vi "Configure Calib Factor (IO).vi"(0 "VISA resource name":refnum<visa-resource-name>, 5 "Channel (0001)":string="0001", 7 "Correct Factor (ON)":bool=TRUE, 9 "Calibration Correction":T1(array[cluster]) {"Sensor Correction Factor" min=-999999 max=999999 step=1; "Instrument Correction Factor" min=-999999 max=999999 step=1; "Uncorrected Value" min=-999999 max=999999 step=1}, 11 "error in (no error)":errorcluster) -> (4 "VISA resource name out":refnum<visa-resource-name>, 6 "Channel":string, 15 "error out":errorcluster)   [LabVIEW 2020, in "Yokogawa GX Series.lvlib"]
doc: "Sets the calibration correction(Correction Factor) for AI channels.\n\nCommand: SCalibIO"
uses:
  <instrlib>/Yokogawa GX Series/Yokogawa GX Series.lvlib
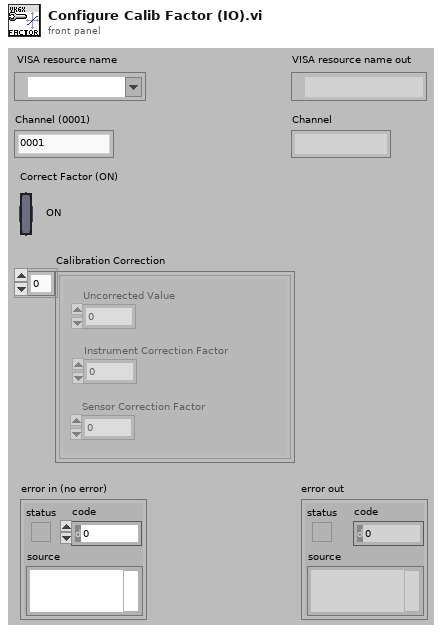
[diagram p1: front panel]
types:
  T1 = cluster{"Uncorrected Value":i32, "Instrument Correction Factor":i32, "Sensor Correction Factor":i32}[]
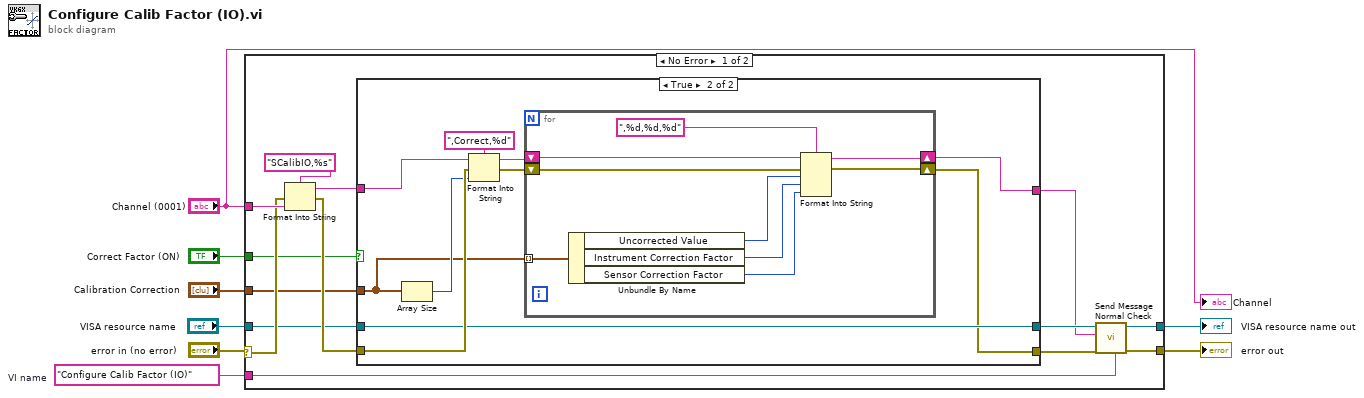
[diagram p0: block diagram]
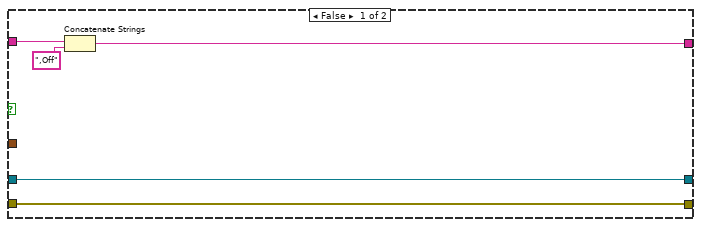
[diagram p2: hidden frame]
diagram:
  w8 = "Configure Calib Factor (IO)"  # VI name
  n1 = case shown="No Error" "error in (no error)" {
    selector: "error in (no error)" -> [w15 w47]
    tunnel: w8 -> [w22 _]
    tunnel: [w21 w48] -> w7
    tunnel: [w20 w47] -> w6
    tunnel: "VISA resource name" -> [w14 w48]
    tunnel: "Channel (0001)" -> [w16 _]
    tunnel: "Correct Factor (ON)" -> [w11 _]
    tunnel: "Calibration Correction" -> [w10 _]
    frame No Error {
      n2 = Format Into String(format string="SCalibIO,%s", error in=w15, w16) -> (resulting string=w18:string, error out=w17:errorcluster)  [unwired: 1 in]
      n3 = case shown="True" w11 {
        tunnel: w18 -> [w27 w29]
        tunnel: [w25 w33] -> w9
        tunnel: w17 -> [w23 w36]
        tunnel: w14 -> [w24 w32]
        tunnel: [w24 w32] -> w13
        tunnel: [w23 w31] -> w12
        tunnel: w10 -> [_ w28]
        frame False {
          n4 = Concatenate Strings(w27, ",Off") -> (w25:string)
        }
        frame True {
          n5 = Array Size(array=w28) -> (size(s)=w30:i32)
          n6 = Format Into String(format string=",Correct,%d", initial string=w29, error in=w36, w30) -> (resulting string=w35:string, error out=w34:errorcluster)
          n7 = for {
            shift-right: [w43] -> w33
            shift-left: w35 -> [w46]
            shift-right: [w44] -> w31
            shift-left: w34 -> [w45]
            tunnel: w28 -> [w40] mode=indexing
            n8 = Unbundle By Name(w40) -> ("Uncorrected Value"=w41:i32, "Instrument Correction Factor"=w39:i32, "Sensor Correction Factor"=w38:i32)
            n9 = Format Into String(format string=",%d,%d,%d", initial string=w46, error in=w45, w41, w39, w38) -> (resulting string=w43:string, error out=w44:errorcluster)
          }
        }
      }
      n10 = call <instrlib>:"Send Message Normal Check.vi"("Source (\"\")"=w22, "error in (no error)"=w12, "Send Message (\"\")"=w9, "VISA resource name"=w13) -> ("error out"=w20:errorcluster, "VISA resource name out"=w21:refnum<visa-resource-name>)  [unwired: 2 in, 4 out]
    }
    frame Error {
    }
  }
  "error out" <- w6
  "VISA resource name out" <- w7
  "Channel" <- "Channel (0001)"
